vi "VISA AMI430 Write-Read.vi"(8 "error in (no error)":errorcluster {"code" format="%.0x"}, 9 "Command String":string="*IDN?", 10 "Action":enum16{"Write", "Read", "Write & Read"}(ring)=enum."Write & Read", 11 "VISA resource name":refnum<visa-resource-name>) -> (0 "error out":errorcluster, 1 "Timeout?":bool, 2 "Response string":string, 3 "dup VISA Session":refnum<visa-resource-name>)   [LabVIEW 2021]
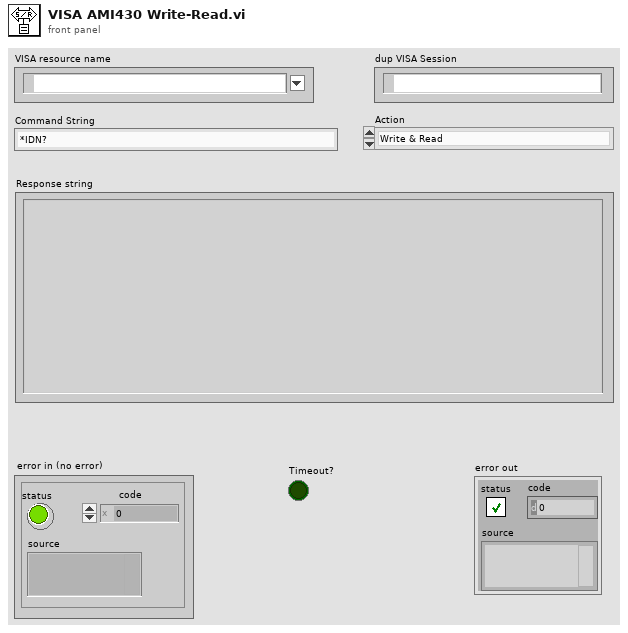
[diagram p1: front panel]
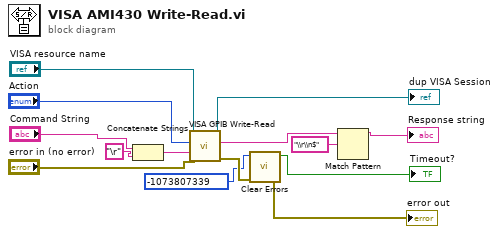
[diagram p0: block diagram]
diagram:
  n1 = Concatenate Strings("Command String", "\r") -> (w3:string)
  n2 = call "VISA GPIB Write-Read.vi"("error in (no error)"="error in (no error)", "Command"=w3, "Action"="Action", "VISA resource name"="VISA resource name") -> ("error out"=w10:errorcluster, "String Returned"=w7:string, "dup VISA Session"=→"dup VISA Session":refnum<visa-resource-name>)  [unwired: 4 in, 1 out]
  n3 = call <vilib>:"Clear Errors.vi"("error in (no error)"=w10, "specific error code to clear (0: all)"=-1073807339) -> ("error out"=→"error out":errorcluster, "specific error cleared?"=→"Timeout?":bool)  [unwired: 4 in]
  n4 = Match Pattern(string=w7, regular expression="\\r\\n$") -> (before substring=→"Response string":string)  [unwired: 1 in, 3 out]
